vi "SVPO Single Block Power Spectrum (N Ch DBL Array).vi"(0 "scaled signal [EU]":dbl[][](array[numeric]), 1 "sampling rate [Hz]":dbl=1.0, 2 "window":T7=1 items=["None"=0, "Hanning"=1, "Hamming"=2, "Blackman-Harris"=3, "Exact Blackman"=4, "Blackman"=5, "Flat Top"=6, "4 Term B-Harris "=7, "7 Term B-Harris"=8, "Low Sidelobe"=9, "Force"=64, "Exponential"=65, "Blackman Nuttall"=11, "Triangle"=30, "Bartlett-Hanning"=31, "Bohman"=32, "Parzen"=33, "Welch"=34, "Kaiser"=60, "Dolph-Chebyshev"=61, "Gaussian"=62]) -> (14 "power spectra [EU^2 rms]":cluster{"f0":dbl, "df":dbl, "magnitude":dbl[]}[](array[cluster]), 18 "spectrum info":T1={"channel name"="", "description"="", "x-axis units"=0, "spectral info"={"spectrum type"=enum."Power [Magnitude^2]", "linear/dB"=enum."linear", "window"=0, "window size"=0, "FFT size"=0}, "engineering units"=1, "custom label"="", "dB reference [EU]"=0.0, "peak units"=enum."rms", "weighting filter"=0, "spectral density?"=FALSE, "unit label"="", "spectrum skewed?"=FALSE, "complimentary spectrum units"=enum."none"} {"x-axis units" items=["Time (s)"=0, "Frequency-CB (Hz)"=1, "Frequency-CPB (Hz)"=1248, "Frequency-Arbitrary (Hz)"=2357, "Quefrency (s)"=2, "Revolutions (rev)"=3, "Order"=4, "Speed (RPM)"=11, "Speed (rad/s)"=21, "Index"=65535]; "weighting filter" items=["Linear", "A-weighting", "B-weighting", "C-weighting", "ITU-R 468-4", "Dolby", "CCITT", "C-message", "Wb", "Wc", "Wd", "We", "Wf", "Wh", "Wj", "Wk", "Wm", "AES17 20 kHz lowpass", "AES17 40 kHz lowpass", "AES17 20 kHz highpass", "AES17 40 kHz highpass"]; "dB reference [EU]" format="%.2f"; "engineering units" items=["custom..."=0, "V"=1, "A"=21, "C"=30, "pC"=31, "s"=32, "-"=29, "Pa"=2, "N"=20, "g"=3, "m/s^2"=4, "m/s"=5, "m"=6, "mm/s"=12, "mm"=13, "micron/s"=14, "micron"=15, "in/s^2"=7, "in/s"=8, "in"=9, "mil/s"=10, "mil"=11, "rad/s^2"=16, "rad/s"=17, "rad"=18, "deg/s^2"=26, "deg/s"=27, "deg"=28, "RPM"=22, "cycle/s^2"=23, "Hz"=24, "cycle"=25, "strain"=19]; "spectral info"."window" items=["None "=0, "Hanning"=1, "Hamming"=2, "Blackman-Harris"=3, "Exact Blackman"=4, "Blackman"=5, "Flat Top"=6, "4 Term B-Harris "=7, "7 Term B-Harris"=8, "Low Sidelobe"=9, "Force - Exponential"=10, "Gaussian"=62]})   [LabVIEW 2017]
doc: "Computes the linear RMS-averaged power spectrum of <B>scaled signal [EU]</B> in a linear scale. Use the power spectrum to quantify signal components as a function of frequency. Use this VI on embedded targets that have limited computational resources. Wire data to the <B>scaled signal [EU]</B> input to determine the polymorphic instance to use or manually select the instance."
uses:
  <vilib>/addons/_NISVFA/_Shared subVIs/Controls/svc_Window.ctl
  <vilib>/addons/_NISVFA/_Shared subVIs/Controls/svc_Spectrum Info.ctl
  <vilib>/addons/_NISVFA/_Shared subVIs/Controls/svc_X-Axis Units.ctl
  <vilib>/addons/_NISVFA/_Shared subVIs/Controls/svc_Spectrum Type.ctl
  <vilib>/addons/_NISVFA/_Shared subVIs/Controls/svc_Engineering Units Text Ring.ctl
  <vilib>/addons/_NISVFA/_Shared subVIs/Controls/svc_Weighting Filter Text Ring.ctl
  <vilib>/addons/_NISVFA/_Shared subVIs/Controls/svc_Complimentary Spectrum Units.ctl
  <vilib>/addons/_NISVFA/_Baseband FFT/subVIs/svfa_Convert to One-Sided Power Spectrum.vi
  <vilib>/Analysis/2dsp.llb/Power Spectrum.vi
  <vilib>/Analysis/2dsp.llb/Power Spectrum (DBL).vi
  <vilib>/addons/_NISVFA/_Shared subVIs/Windowing/svfa_Scaled Time Domain Window (Array).vi
  <vilib>/Analysis/4window.llb/Force Window.vi
  <vilib>/Analysis/4window.llb/Force Window (DBL).vi
  <vilib>/Analysis/4window.llb/Exponential Window.vi
  <vilib>/Analysis/4window.llb/Exponential Window (DBL).vi
  <vilib>/Utility/error.llb/Error Cluster From Error Code.vi
  <vilib>/Analysis/0measdsp.llb/Scaled Time Domain Window.vi
  <vilib>/Analysis/0measdsp.llb/Scaled Time Domain Window (DBL).vi
  <vilib>/addons/_NISVFA/_Spectrum Processing/subVIs/svfa_Spectrum Info Window to windowTd Type Def.vi
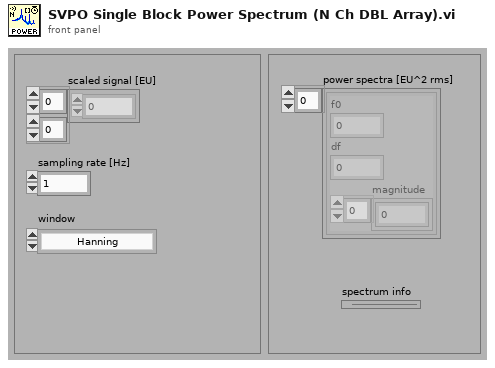
[diagram p1: front panel]
types:
  T1 = typedef "svc_Spectrum Info.ctl" = cluster{"channel name":string, "description":string, "x-axis units":T2, "spectral info":cluster{"spectrum type":T3, "linear/dB":enum16{"linear", "dB"}, "window":u16, "window size":i32, "FFT size":i32}, "engineering units":T4, "custom label":string, "dB reference [EU]":dbl, "peak units":enum16{"rms", "peak", "peak-peak"}, "weighting filter":T5, "spectral density?":bool, "unit label":string, "spectrum skewed?":bool, "complimentary spectrum units":T6}
  T2 = typedef "svc_X-Axis Units.ctl" = u16
  T3 = typedef "svc_Spectrum Type.ctl" = enum16{"FFT Spectrum [complex]", "Amplitude [Magnitude]", "Power [Magnitude^2]", "Cross Spectrum [complex]", "Frequency Response [Complex]"}
  T4 = typedef "svc_Engineering Units Text Ring.ctl" = u16
  T5 = typedef "svc_Weighting Filter Text Ring.ctl" = u16
  T6 = typedef "svc_Complimentary Spectrum Units.ctl" = enum16{"none", "radians", "degrees", "cycles", "imaginary"}
  T7 = typedef "svc_Window.ctl" = u32
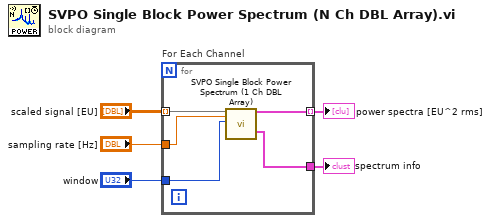
[diagram p0: block diagram]
diagram:
  n1 = for "For Each Channel" {
    tunnel: "window" -> [w9]
    tunnel: "scaled signal [EU]" -> [w10] mode=indexing
    tunnel: "sampling rate [Hz]" -> [w8]
    tunnel: [w6] -> w1
    tunnel: [w7] -> w2 mode=indexing
    n2 = call <vilib>:"SVPO Single Block Power Spectrum (1 Ch DBL Array).vi"("scaled signal [EU]"=w10, "sampling rate [Hz]"=w8, "window"=w9) -> ("power spectrum [EU^2 rms]"=w7:cluster{"f0":dbl, "df":dbl, "magnitude":dbl[]}, "spectrum info"=w6:T1)  [unwired: 15 in]
  }
  "power spectra [EU^2 rms]" <- w2
  "spectrum info" <- w1
